vi "Get time series list.vi"(0 "InfluxDB in":refnum<class "InfluxDB Client.lvclass">, 5 "Database name":string, 11 "error in (no error)":errorcluster) -> (4 "InfluxDB out":refnum<class "InfluxDB Client.lvclass">, 6 "Time series names":string[](array[string]), 15 "error out":errorcluster)   [LabVIEW 2017]
doc: "Gets a list of available time series within a database."
uses:
  <vilib>/httpClient/LabVIEWHTTPClient.lvlib
  InfluxDB Client.lvclass
  <vilib>/LVH/i3 JSON/i3-json.lvlib
  <vilib>/LVH/i3 JSON/JSON Parsing/Get Object Parameter Files/Get Object Parameter - Array.vi
  <vilib>/LVH/i3 JSON/JSON Parsing/Get Array Value at Index Files/Get Array Value at Index - Array.vi
  <vilib>/LVH/i3 JSON/JSON Parsing/Get Array Value at Index Files/Get Array Value at Index - String.vi
  <vilib>/LVH/i3 JSON/JSON Parsing/Get Array Value at Index Files/Get Array Value at Index - Object.vi
panel:
  out "Status":string
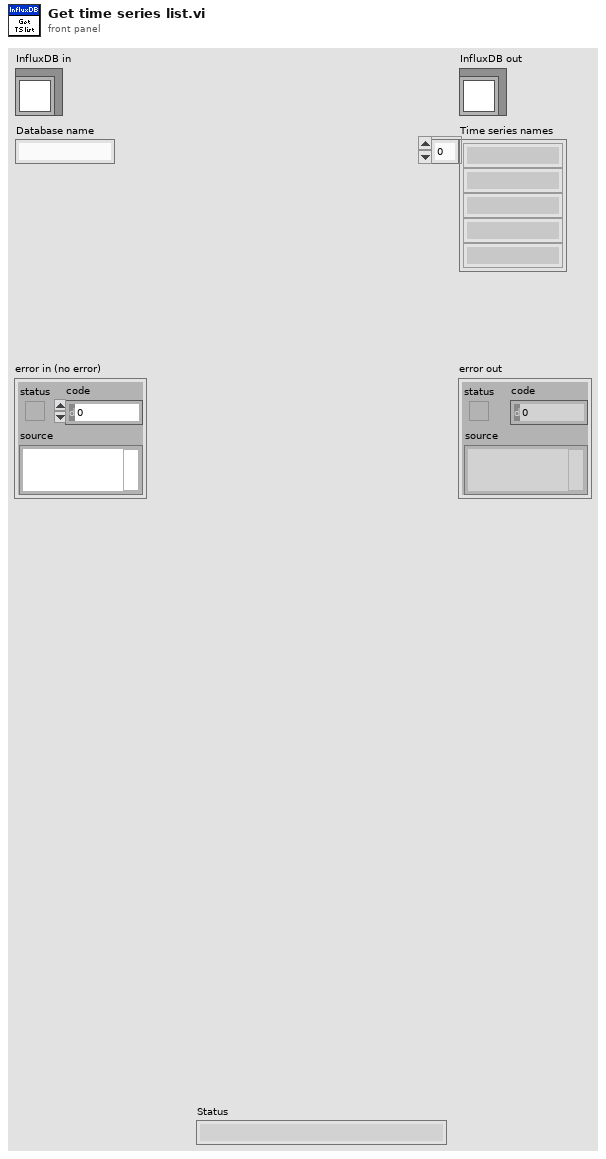
[diagram p1: front panel]
types:
  T1 = typedef "LabVIEWHTTPClient.lvlib/ClientHandle.ctl" = refnum<k1>
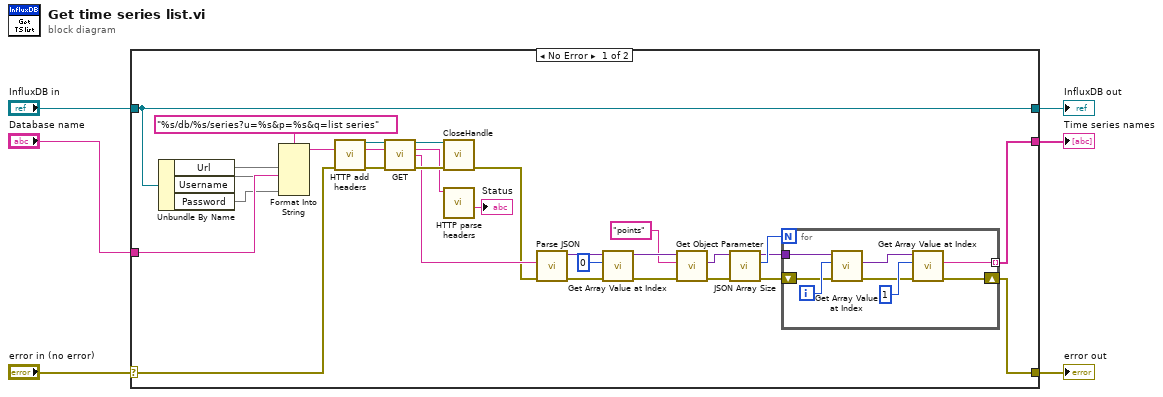
[diagram p0: block diagram]
diagram:
  n1 = case shown="No Error" "error in (no error)" {
    selector: "error in (no error)" -> [w24 w45]
    tunnel: [w7 w45] -> w5
    tunnel: [w35 w44] -> w3
    tunnel: "InfluxDB in" -> [w35 w44]
    tunnel: [w13 _] -> w2
    tunnel: "Database name" -> [w27 _]
    frame No Error {
      n2 = Unbundle By Name(w35) -> ("Url"=w33, "Username"=w26, "Password"=w25)
      n3 = Format Into String(format string="%s/db/%s/series?u=%s&p=%s&q=list series" ("url"), w33, w27, w26, w25) -> (resulting string=w30:string)  [unwired: 2 in, 1 out]
      n4 = call "HTTP add headers.vi"("error in (no error)"=w24) -> ("client handle out"=w23:T1, "error out"=w22:errorcluster)  [unwired: 13 in]
      n5 = call <vilib>:"GET.vi"("client handle"=w23, "url"=w30, "error in (no error)"=w22) -> ("client handle out"=w32:T1, "headers"=w29:string, "body"=w14:string, "error out"=w31:errorcluster)  [unwired: 9 in]
      n6 = call <vilib>:"CloseHandle.vi"("client handle"=w32, "error in (no error)"=w31) -> ("error out"=w12:errorcluster)  [unwired: 13 in]
      n7 = call "HTTP parse headers.vi"("HTTP headers"=w29) -> ("Status"=→"Status":string)  [unwired: 8 in, 2 out]
      n8 = call <vilib>:"Parse JSON.vi"("error in (no error)"=w12, "JSON String"=w14) -> ("error out"=w11:errorcluster, "JSON Tree"=w15:variant)  [unwired: 6 in, 2 out]
      n9 = call-poly <vilib>:"Get Array Value at Index.vi"("error in (no error)"=w11, "Index"=0, "JSON Tree In (JSON Array)"=w15) -> ("error out"=w10:errorcluster, "JSON Object"=w21:variant)  [unwired: 5 in, 2 out]
      n10 = call-poly <vilib>:"Get Object Parameter.vi"("error in (no error)"=w10, "Parameter Name"="points", "JSON Tree In (JSON Object)"=w21) -> ("error out"=w9:errorcluster, "JSON Array"=w17:variant)  [unwired: 5 in, 2 out]
      n11 = call <vilib>:"JSON Array Size.vi"("error in (no error)"=w9, "JSON Tree In (JSON Array)"=w17) -> ("error out"=w8:errorcluster, "Array Size"=w19:i32, "JSON Tree Passthrough (JSON Array)"=w18:variant)  [unwired: 7 in]
      n12 = for {
        N: w19 -> [_]
        tunnel: w18 -> [w43]
        tunnel: [w40] -> w13 mode=indexing
        shift-right: [w36] -> w7
        shift-left: w8 -> [w38]
        i -> [w42]
        n13 = call-poly <vilib>:"Get Array Value at Index.vi"("error in (no error)"=w38, "Index"=w42, "JSON Tree In (JSON Array)"=w43) -> ("error out"=w37:errorcluster, "JSON Array"=w39:variant)  [unwired: 5 in, 2 out]
        n14 = call-poly <vilib>:"Get Array Value at Index.vi"("error in (no error)"=w37, "Index"=1, "JSON Tree In (JSON Array)"=w39) -> ("error out"=w36:errorcluster, "String Value"=w40:string)  [unwired: 5 in, 2 out]
      }
    }
    frame Error {
    }
  }
  "error out" <- w5
  "InfluxDB out" <- w3
  "Time series names" <- w2
